vi "CAN_ReadBMS.vi"(8 "error in (no error)":errorcluster) -> (0 "error out":errorcluster={"status"=TRUE, "code"=-61201, "source"="niLvFpga_Open_cRIO-9063.vi:6100001"})   [LabVIEW 2018]
uses:
  BMS/Orion_BMS.lvclass
  BMS/Orion_BMS.lvclass/Orion_BMS.ctl
  TypeDef_LoopPeriods.ctl
  <vilib>/Platform/TimedLoop/XDataNode/timing_clust.ctl
  <vilib>/Platform/TimedLoop/XDataNode/nitl_modes.ctl
  <vilib>/Platform/TimedLoop/XDataNode/wakeup.ctl
  Control/TypeDef_DigitalOuts.ctl
  TypeDef_BMSData.ctl
  TypeDef_BMS_Status.ctl
  <vilib>/platform/TimedLoop/XDataNode/XDataNode.xnode
  <vilib>/Platform/TimedLoop/XDataNode/XDNodeRunTimeDep.lvlib
panel:
  out "deviceFroze":bool
  out "loopCounter":i32
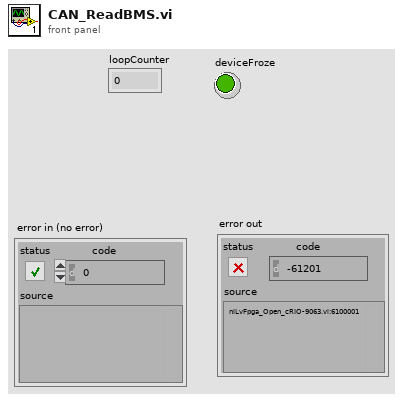
[diagram p1: front panel]
types:
  T1 = typedef "TypeDef_LoopPeriods.ctl" = cluster{"Control Period":i64, "DAQ Period":u32, "IMU Period":u32, "CAN Period":i64, "Nav Period":u32}
  T2 = typedef "XDNodeRunTimeDep.lvlib/timing_clust.ctl" = cluster{"Expected End [f-1]":u64, "Actual End [f-1]":u64, "Finished Late? [f-1]":bool, "Expected End [i-1]":u64, "Actual End [i-1]":u64, "Finished Late? [i-1]":bool, "Expected Start [i]":u64, "Actual Start [i]":u64, "Expected Start [f]":u64, "Actual Start [f]":u64, "Source Name":string, "Structure Name":string, "Period":i64, "Deadline":i64, "Offset":i64, "Start":i64, "Priority":i32, "Timeout":i32, "Mode":T3, "Wakeup Reason":T4, "Error":errorcluster, "Source Type":string, "Secondary Source Type":string, "Global End Time":u64, "Global Start Time":u64, "Frame Duration":u64, "Iteration Duration":u64, "Assigned CPU":i32, "I/O Scan Engine Mode":u32}
  T3 = typedef "XDNodeRunTimeDep.lvlib/nitl_modes.ctl" = enum32{"No Change", "Process missed periods, maintain original phase", "Discard missed periods, maintain original phase", "Process missed periods, ignore original phase", "Discard missed periods, ignore original phase"}
  T4 = typedef "XDNodeRunTimeDep.lvlib/wakeup.ctl" = enum32{"Normal", "Aborted", "Asynchronous wakeup", "Timing source error", "Timed loop error", "Timeout"}
  T5 = typedef "TypeDef_DigitalOuts.ctl" = cluster{"Pod Power":bool, "Dump Valve":bool, "Brakes":bool, "Clamp":bool, "Pump":bool, "Ignition":bool, "DO6":bool, "DO7":bool, "HighSide":bool, "Precharge":bool, "LowSide":bool, "DO3":bool, "DO4":bool, "DO5":bool, "DO62":bool, "DO72":bool}
  T6 = typedef "TypeDef_BMSData.ctl" = cluster{"Max Cell Voltage (V)":dbl, "Max Cell ID":dbl, "Min Cell Voltage (V)":dbl, "Min Cell ID":dbl, "State of Charge (%)":dbl, "Average Voltage (V)":dbl, "Voltage Delta (V)":dbl, "Pack Current (A)":dbl, "Pack Voltage (V)":dbl, "Max Resistance (Ohm)":dbl, "Min Resistance (Ohm)":dbl, "Average Resistance (Ohm)":dbl, "Delta Resistance (Ohm)":dbl, "Highest Temperature(F)":dbl, "BmsStatus":T7}
  T7 = typedef "TypeDef_BMS_Status.ctl" = cluster{"isFault":bool, "isolationMonitoring":bool}
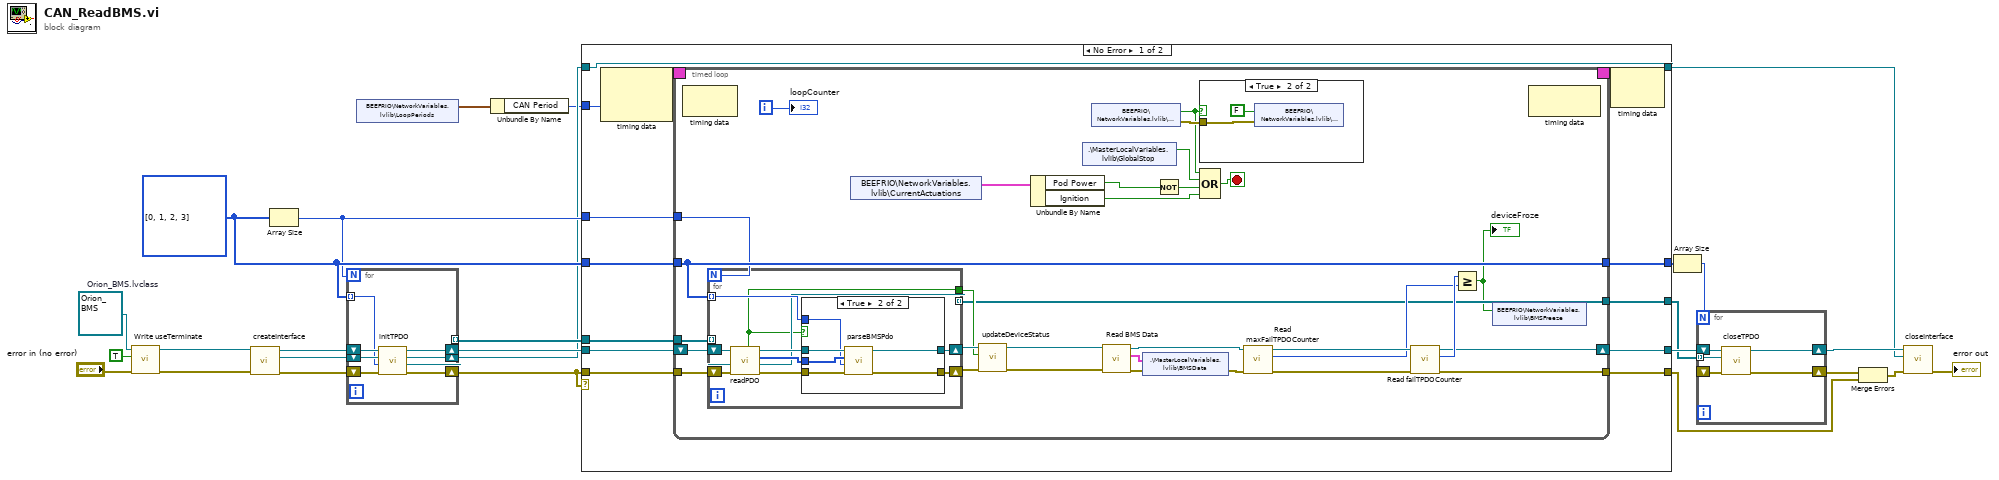
[diagram p0: block diagram]
diagram:
  w3 = refnum<class "Orion_BMS.lvclass"> refnum  # Orion_BMS.lvclass
  w24 = u8[] [0, 1, 2, 3] items=["PDO 1", "PDO 2", "PDO 3", "PDO 4"]
  n1 = call "Write useTerminate.vi"("error in (no error)"="error in (no error)", "useTerminate"=TRUE, "Orion_BMS in"=w3) -> ("error out"=w5:errorcluster, "Orion_BMS out"=w6:refnum<class "Orion_BMS.lvclass">)  [unwired: 7 in]
  n2 = call "createInterface.vi"("error in (no error)"=w5, "Orion_BMS in"=w6) -> ("error out"=w12:errorcluster, "interface object out"=w13:refnum<k20>, "Orion_BMS out"=w14:refnum<class "Orion_BMS.lvclass">)  [unwired: 7 in]
  n3 = Array Size(array=w24) -> (size(s)=w19:i32)
  n4 = for {
    N: w19 -> [_]
    tunnel: w24 -> [w31] mode=indexing
    shift-right: [w28] -> w10
    shift-left: w13 -> [w32]
    tunnel: [w27] -> w25 mode=indexing
    shift-right: [w29] -> w26
    shift-left: w14 -> [w34]
    shift-right: [w30] -> w1
    shift-left: w12 -> [w33]
    n5 = call "initTPDO.vi"("error in (no error)"=w33, "PDO channel"=w31, "interface object in"=w32, "Orion_BMS in"=w34) -> ("error out"=w30:errorcluster, "interface object out"=w28:refnum<k20>, "TPDO object out"=w27:refnum<k20>, "Orion_BMS out"=w29:refnum<class "Orion_BMS.lvclass">)  [unwired: 4 in]
  }
  n6 = shared-variable "BEEFRIO\\NetworkVariables.lvlib\\LoopPeriods"() -> (w8:T1)  [unwired: 1 in, 1 out]
  n7 = Unbundle By Name(w8) -> ("CAN Period"=w7:i64)
  n8 = case shown="No Error" w1 {
    tunnel: w26 -> [w45 w109]
    tunnel: w25 -> [w44 w108]
    tunnel: w24 -> [w43 w110]
    tunnel: [w42 w110] -> w22
    tunnel: [w41 w109] -> w21
    tunnel: [w40 w108] -> w20
    tunnel: w19 -> [w39 _]
    tunnel: [w38 w107] -> w11
    tunnel: w1 -> [w37 w107]
    tunnel: w10 -> [w36 w106]
    tunnel: [w36 w106] -> w9
    tunnel: w7 -> [w35 _]
    frame No Error {
      n9 = node-c288(w35) -> (w47:T2)  [unwired: 1 in]
      n10 = timed-loop {
        timing: w47 -> [_]
        timing-out: [_] -> w46
        tunnel: w44 -> [w77]
        tunnel: w43 -> [w61]
        tunnel: [w62] -> w40
        tunnel: [w61] -> w42
        tunnel: w39 -> [w60]
        shift-right: [w63] -> w41
        shift-left: w45 -> [w78]
        tunnel: [w50] -> w38
        tunnel: w37 -> [w49]
        i -> [w59]
        stop <- w57 stop-if-true
        n11 = node-c288() -> ()  [unwired: 1 in, 1 out]
        n12 = for {
          N: w60 -> [_]
          shift-right: [w83] -> w76
          shift-left: w49 -> [w88]
          tunnel: w77 -> [w86] mode=indexing
          tunnel: w61 -> [w85] mode=indexing
          shift-right: [w84] -> w75
          shift-left: w78 -> [w87]
          tunnel: [w81] -> w74
          tunnel: [w82] -> w62 mode=indexing
          n13 = call "readPDO.vi"("error in (no error)"=w88, "TPDO object in"=w86, "Orion_BMS in"=w87) -> ("error out"=w91:errorcluster, "TPDO object out"=w82:refnum<k20>, "TPDO data"=w90:u8[], "Orion_BMS out"=w89:refnum<class "Orion_BMS.lvclass">, "new data?"=w81:bool)  [unwired: 4 in]
          n14 = case shown="True" w81 {
            tunnel: w91 -> [w92 w99]
            tunnel: w90 -> [_ w98]
            tunnel: w89 -> [w93 w97]
            tunnel: w85 -> [_ w96]
            tunnel: [w93 w95] -> w84
            tunnel: [w92 w94] -> w83
            frame False {
            }
            frame True {
              n15 = call "parseBMSPdo.vi"("error in (no error)"=w99, "PDO channel"=w96, "TPDO data"=w98, "Orion_BMS in"=w97) -> ("error out"=w94:errorcluster, "Orion_BMS out"=w95:refnum<class "Orion_BMS.lvclass">)  [unwired: 6 in]
            }
          }
        }
        n16 = shared-variable "BEEFRIO\\NetworkVariables.lvlib\\CurrentActuations"() -> (w56:T5)  [unwired: 1 in, 1 out]
        n17 = call "updateDeviceStatus.vi"("error in (no error)"=w76, "isNewData"=w74, "Orion_BMS in"=w75) -> ("error out"=w66:errorcluster, "Orion_BMS out"=w65:refnum<class "Orion_BMS.lvclass">)  [unwired: 7 in]
        n18 = Unbundle By Name(w56) -> ("Pod Power"=w55:bool, "Ignition"=w48:bool)
        n19 = shared-variable ".\\MasterLocalVariables.lvlib\\GlobalStop"() -> (w53:bool)  [unwired: 1 in, 1 out]
        n20 = shared-variable "BEEFRIO\\NetworkVariables.lvlib\\ReintCAN"() -> (w51:bool, error out=w52:errorcluster)  [unwired: 1 in]
        n21 = call "Read BMS Data.vi"("error in (no error)"=w66, "Orion_BMS in"=w65) -> ("error out"=w72:errorcluster, "BMS Data"=w71:T6, "Orion_BMS out"=w67:refnum<class "Orion_BMS.lvclass">)  [unwired: 7 in]
        n22 = shared-variable ".\\MasterLocalVariables.lvlib\\BMSData"(w71, error in=w72) -> (error out=w73:errorcluster)
        n23 = Not(x=w55) -> (.not. x?=w54:bool)
        n24 = case shown="True" w51 {
          tunnel: w52 -> [_ w80]
          frame False {
          }
          frame True {
            n25 = shared-variable "BEEFRIO\\NetworkVariables.lvlib\\ReintCAN"(FALSE ("ReintCAN"), error in=w80) -> ()  [unwired: 1 out]
          }
        }
        n26 = Compound Arithmetic op=OR(w51, w53, w54, w48) -> (w57:bool)
        n27 = call "Read maxFailTPDOCounter.vi"("error in (no error)"=w73, "Orion_BMS in"=w67) -> ("error out"=w69:errorcluster, "maxFailTPDOCounter"=w64:u8, "Orion_BMS out"=w68:refnum<class "Orion_BMS.lvclass">)  [unwired: 7 in]
        n28 = call "Read failTPDOCounter.vi"("error in (no error)"=w69, "Orion_BMS in"=w68) -> ("error out"=w50:errorcluster, "failTPDOCounter"=w70:u32, "Orion_BMS out"=w63:refnum<class "Orion_BMS.lvclass">)  [unwired: 7 in]
        n29 = Greater Or Equal?(x=w70, y=w64) -> (x >= y?=w58:bool)
        "deviceFroze" <- w58
        n30 = shared-variable "BEEFRIO\\NetworkVariables.lvlib\\BMSFreeze"(w58) -> ()  [unwired: 1 in, 1 out]
        n31 = node-c288() -> ()  [unwired: 1 in, 1 out]
        "loopCounter" <- w59
      }
      n32 = node-c288(w46) -> ()  [unwired: 1 out]
    }
    frame Error {
    }
  }
  n33 = Array Size(array=w22) -> (size(s)=w23:i32)
  n34 = for {
    N: w23 -> [_]
    shift-right: [w111] -> w16
    shift-left: _ -> [w115]
    shift-right: [w113] -> w18
    shift-left: w21 -> [w114]
    tunnel: w20 -> [w112] mode=indexing
    n35 = call "closeTPDO.vi"("error in (no error)"=w115, "TPDO object in"=w112, "Orion_BMS in"=w114) -> ("error out"=w111:errorcluster, "Orion_BMS out"=w113:refnum<class "Orion_BMS.lvclass">)  [unwired: 7 in]
  }
  n36 = Merge Errors(w16, w11) -> (w15:errorcluster)
  n37 = call "closeInterface.vi"("error in (no error)"=w15, "interface object in"=w9, "Orion_BMS in"=w18) -> ("error out"=→"error out":errorcluster)  [unwired: 7 in, 1 out]
